vi "Compute (Array).vi"(8 "error in (no error)":errorcluster, 10 "Data Points in":T1, 11 "Normalize in":refnum<class "Normalize.lvclass">) -> (0 "error out":errorcluster, 2 "Data Points out":T1, 3 "Normalize out":refnum<class "Normalize.lvclass">)   [LabVIEW 2017, in "Normalize.lvclass"]
doc: "Process and return an array of data points at the end of a scan. (For example, to normalize the output or find min/max, one must know all data points a priori.)"
uses:
  Normalize.lvclass
  Instruments/Utility Classes/Readable/Data Points.ctl
  Instruments/Utility Classes/Readable/Data Point.ctl
  Instruments/Utility Classes/Readable/Time.ctl
  Instruments/Utility Classes/Readable/X.ctl
  <vilib>/Analysis/baseanly.llb/Normalize Vector.vi
  <vilib>/Analysis/NI_AALBase.lvlib
  Instruments/Utility Classes/Readable/Readable.lvclass
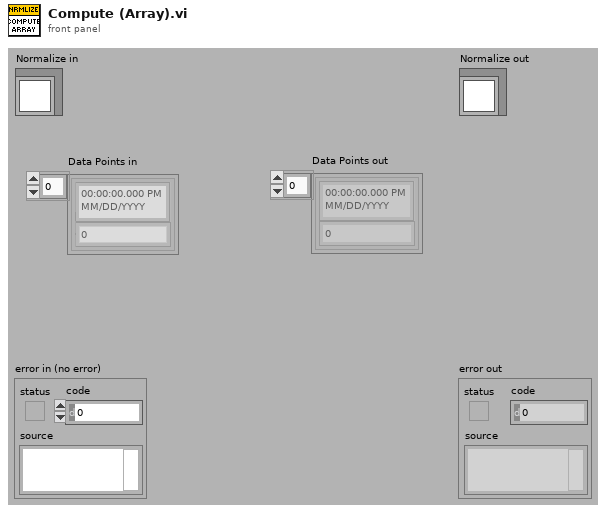
[diagram p1: front panel]
types:
  T1 = typedef "Readable.lvclass/Data Points.ctl" = T2[]
  T2 = typedef "Readable.lvclass/Data Point.ctl" = cluster{"t":T3, "x":T4}
  T3 = typedef "Readable.lvclass/Time.ctl" = timestamp
  T4 = typedef "Readable.lvclass/X.ctl" = dbl
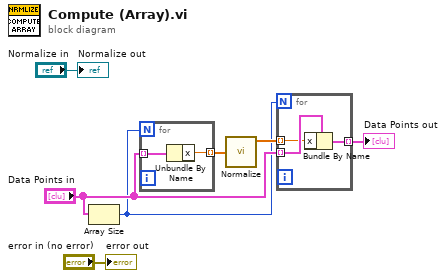
[diagram p0: block diagram]
diagram:
  n1 = Array Size(array="Data Points in") -> (size(s)=w1:i32)
  n2 = for {
    N: w1 -> [_]
    tunnel: "Data Points in" -> [w9] mode=indexing
    tunnel: [w8] -> w5 mode=indexing
    n3 = Unbundle By Name(w9) -> ("x"=w8:T4)
  }
  n4 = call-poly <vilib>:"Normalize.vi"("Vector"=w5) -> ("Normalized Vector"=w4:dbl[])  [unwired: 1 in, 3 out]
  n5 = for {
    N: w1 -> [_]
    tunnel: w4 -> [w11] mode=indexing
    tunnel: "Data Points in" -> [w12] mode=indexing
    tunnel: [w10] -> w3 mode=indexing
    n6 = Bundle By Name(cluster=w12, "x"=w11) -> (w10:T2)
  }
  "Data Points out" <- w3
  "error out" <- "error in (no error)"
  "Normalize out" <- "Normalize in"
